vi "UiControls_b2g2.vi"() -> ()   [LabVIEW 2011]
uses:
  Output - Cluster b2g2.ctl
  Input - Cluster b2g2.ctl
panel:
  out "Array":errorcluster[](array[cluster])
  in  "Tab Control":enum32{"auto", "manual", "timetable", "tools"}(tab)
  in  "circulation ctl":bool
  in  "off [min]":u8=10 step=1 format="%#_3g"
  in  "on [min]":u8=10 step=1 format="%#_3g"
  in  "level ctl":bool
  in  "pressure ctl":bool
  in  "dosage ctl":bool
  in  "temp. ctl":bool
  in  "setpoint [l]":sgl=2.4 min=0 max=5 step=0.1 format="%.1g"
  in  "setpoint [bar]":sgl=10.0 min=0 max=10 step=0.1 format="%.1g"
  in  "flow [l/min]":sgl=1.5 format="%.1g"
  in  "volume [l]":sgl=1.0 step=0.1 format="%.1g"
  in  "hysteresis [°C]":sgl=0.05 min=0.01 max=10 step=0.01 format="%.2g"
  in  "setpoint [°C]":sgl=37.0 min=0 max=100 step=0.1 format="%.1g"
  in  "Tank":enum32{"Tank 1", "Tank 2 (Flash)"}(radio) caption="source"
  in  "P-9":bool
  in  "V-34":bool
  in  "V-33":bool
  in  "V-13 [%]":u8=10 caption="opening [%]" max=100 step=1
  in  "V-15  [%]":u8 caption="opening [%]" max=100 step=1
  in  "P-4 Drehzahl  [%]":u8=50 caption="speed  [%]"
  in  "P-4":bool
  in  "HS-1":bool
  in  "Interval [ms]":u32=10 caption="interval [ms]" min=10 step=1
  in  "Target Log":bool caption="crio log"
  in  "V-35":bool
  in  "T-1 & T-2  \nlevel-monitoring":bool=TRUE
  in  "MR \nlevel-monitoring":bool=TRUE
  out "Volume T-2 [l]":dbl caption="T-2 [l]"
  out "Volume T-1 [l]":dbl caption="T-1 [l]"
  in  "on/off":bool caption="activate"
  in  "Zeitplan":string[][](table)=[["00:00", "0", "1", "1", "1,5"], ["01:00", "0", "1", "1", "1,5"], ["02:00", "0", "1", "1", "1,5"], ["03:00", "0", "1", "1", "1,5"], ["04:00", "0", "1", "1", "1,5"], ["05:00", "0", "1", "1", "1,5"], ["06:00", "0", "1", "1", "1,5"], ["07:00", "0", "1", "1", "1,5"], ["08:00", "0", "1", "1", "1,5"], ["09:00", "0", "1", "1", "1,5"], ["10:00", "0", "1", "1", "1,5"], ["11:00", "0", "1", "1", "1,5"], ["12:00", "0", "1", "1", "1,5"], ["13:00", "0", "1", "1", "1,5"], ["14:00", "0", "1", "1", "1,5"], ["15:00", "0", "1", "1", "1,5"], ["16:00", "0", "1", "1", "1,5"], ["17:00", "0", "1", "1", "1,5"], ["18:00", "0", "1", "1", "1,5"], ["19:00", "0", "1", "1", "1,5"], ["20:00", "0", "1", "1", "1,5"], ["21:00", "0", "1", "1", "1,5"], ["22:00", "0", "1", "1", "1,5"], ["23:00", "0", "1", "1", "1,5"]]
  in  "stop":bool caption="stop crio"
  out "pc":timestamp
  out "crio":timestamp
  in  "load/save":enum16{"Load", "Save"}(ring)
  in  "enter":bool
  in  "config file":path caption="path"
  # "accumulated \nvolume"
  # "timestamp"
  # "configurtaion file"
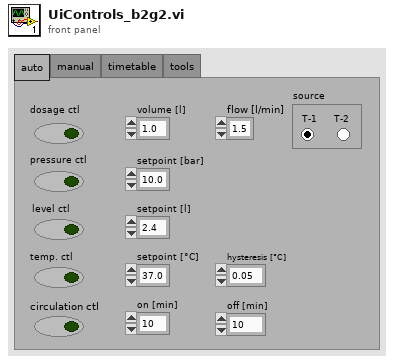
[diagram p1: front panel]
types:
  T1 = typedef "Output - Cluster b2g2.ctl" = cluster{"DFS-1 [dl]":u64, "FS-3 [l]":dbl, "DFS-1 [l/min]":dbl, "DS-1 [bar]":dbl, "V-10 ZU":bool, "V-14 ZU":bool, "FS-1 [l]":dbl, "FS-2 [l]":dbl, "TS-4 [°C]":dbl, "HS-1":bool, "V-13 [%]":u8, "V-15 [%]":u8, "P-4 [%]":u8, "Dosierung":bool, "MR Max Füllstand":bool, "MR Min Füllstand":bool, "Dosiermenge [l]":sgl, "V-14 AUF":bool, "V-10 AUF":bool, "T-1 Max Füllstand":bool, "T-1 Min Füllstand":bool, "T-2 Max Füllstand":bool, "T-2 Min Füllstand":bool, "pHS-1 [pH]":dbl, "P-4 RUN":bool, "V-33 AUF":bool, "V-33 ZU":bool, "V-34 AUF":bool, "V-34 ZU":bool, "P-4 ERR":bool, "TS-5 [°C]":dbl, "V-35 AUF":bool, "V-35 ZU":bool, "P-9 RUN":bool}
  T2 = typedef "Input - Cluster b2g2.ctl" = cluster{"V-13 [%]":u8, "V-15 [%]":u8, "Log-Target":bool, "P-4":bool, "P-4 Drehzahl [%]":u8, "Temperaturregelung":bool, "Überdruckregelung":bool, "Füllstandsregulierung":bool, "V-10":bool, "Log-Host":bool, "V-14":bool, "HS-1":bool, "Füllstand  P":sgl, "Füllstand I":sgl, "Füllstand D":sgl, "Füllstand Soll [l]":sgl, "Druck  P":sgl, "Druck I":sgl, "Druck D":sgl, "Druck Soll [bar]":sgl, "Temp Soll [°C]":sgl, "Dosierung":bool, "Dosiermenge [l]":sgl, "Dosiergeschw. [l/min]":sgl, "Tank":bool, "Hysterese [°C]":sgl, "MR Füllstandsüberwachung":bool, "Tank Füllstandsüberwachung":bool, "Log Target [ms]":u32, "Log Host [s]":u32, "Zirkulation EIN [min]":u8, "Zirkulation AUS [min]":u8, "Zirkulation":bool, "V-33":bool, "V-34":bool, "V-35":bool, "T1 Max Füllstand":bool, "T1 Min Füllstand":bool, "FS-1 [l]":sgl, "P-9":bool}
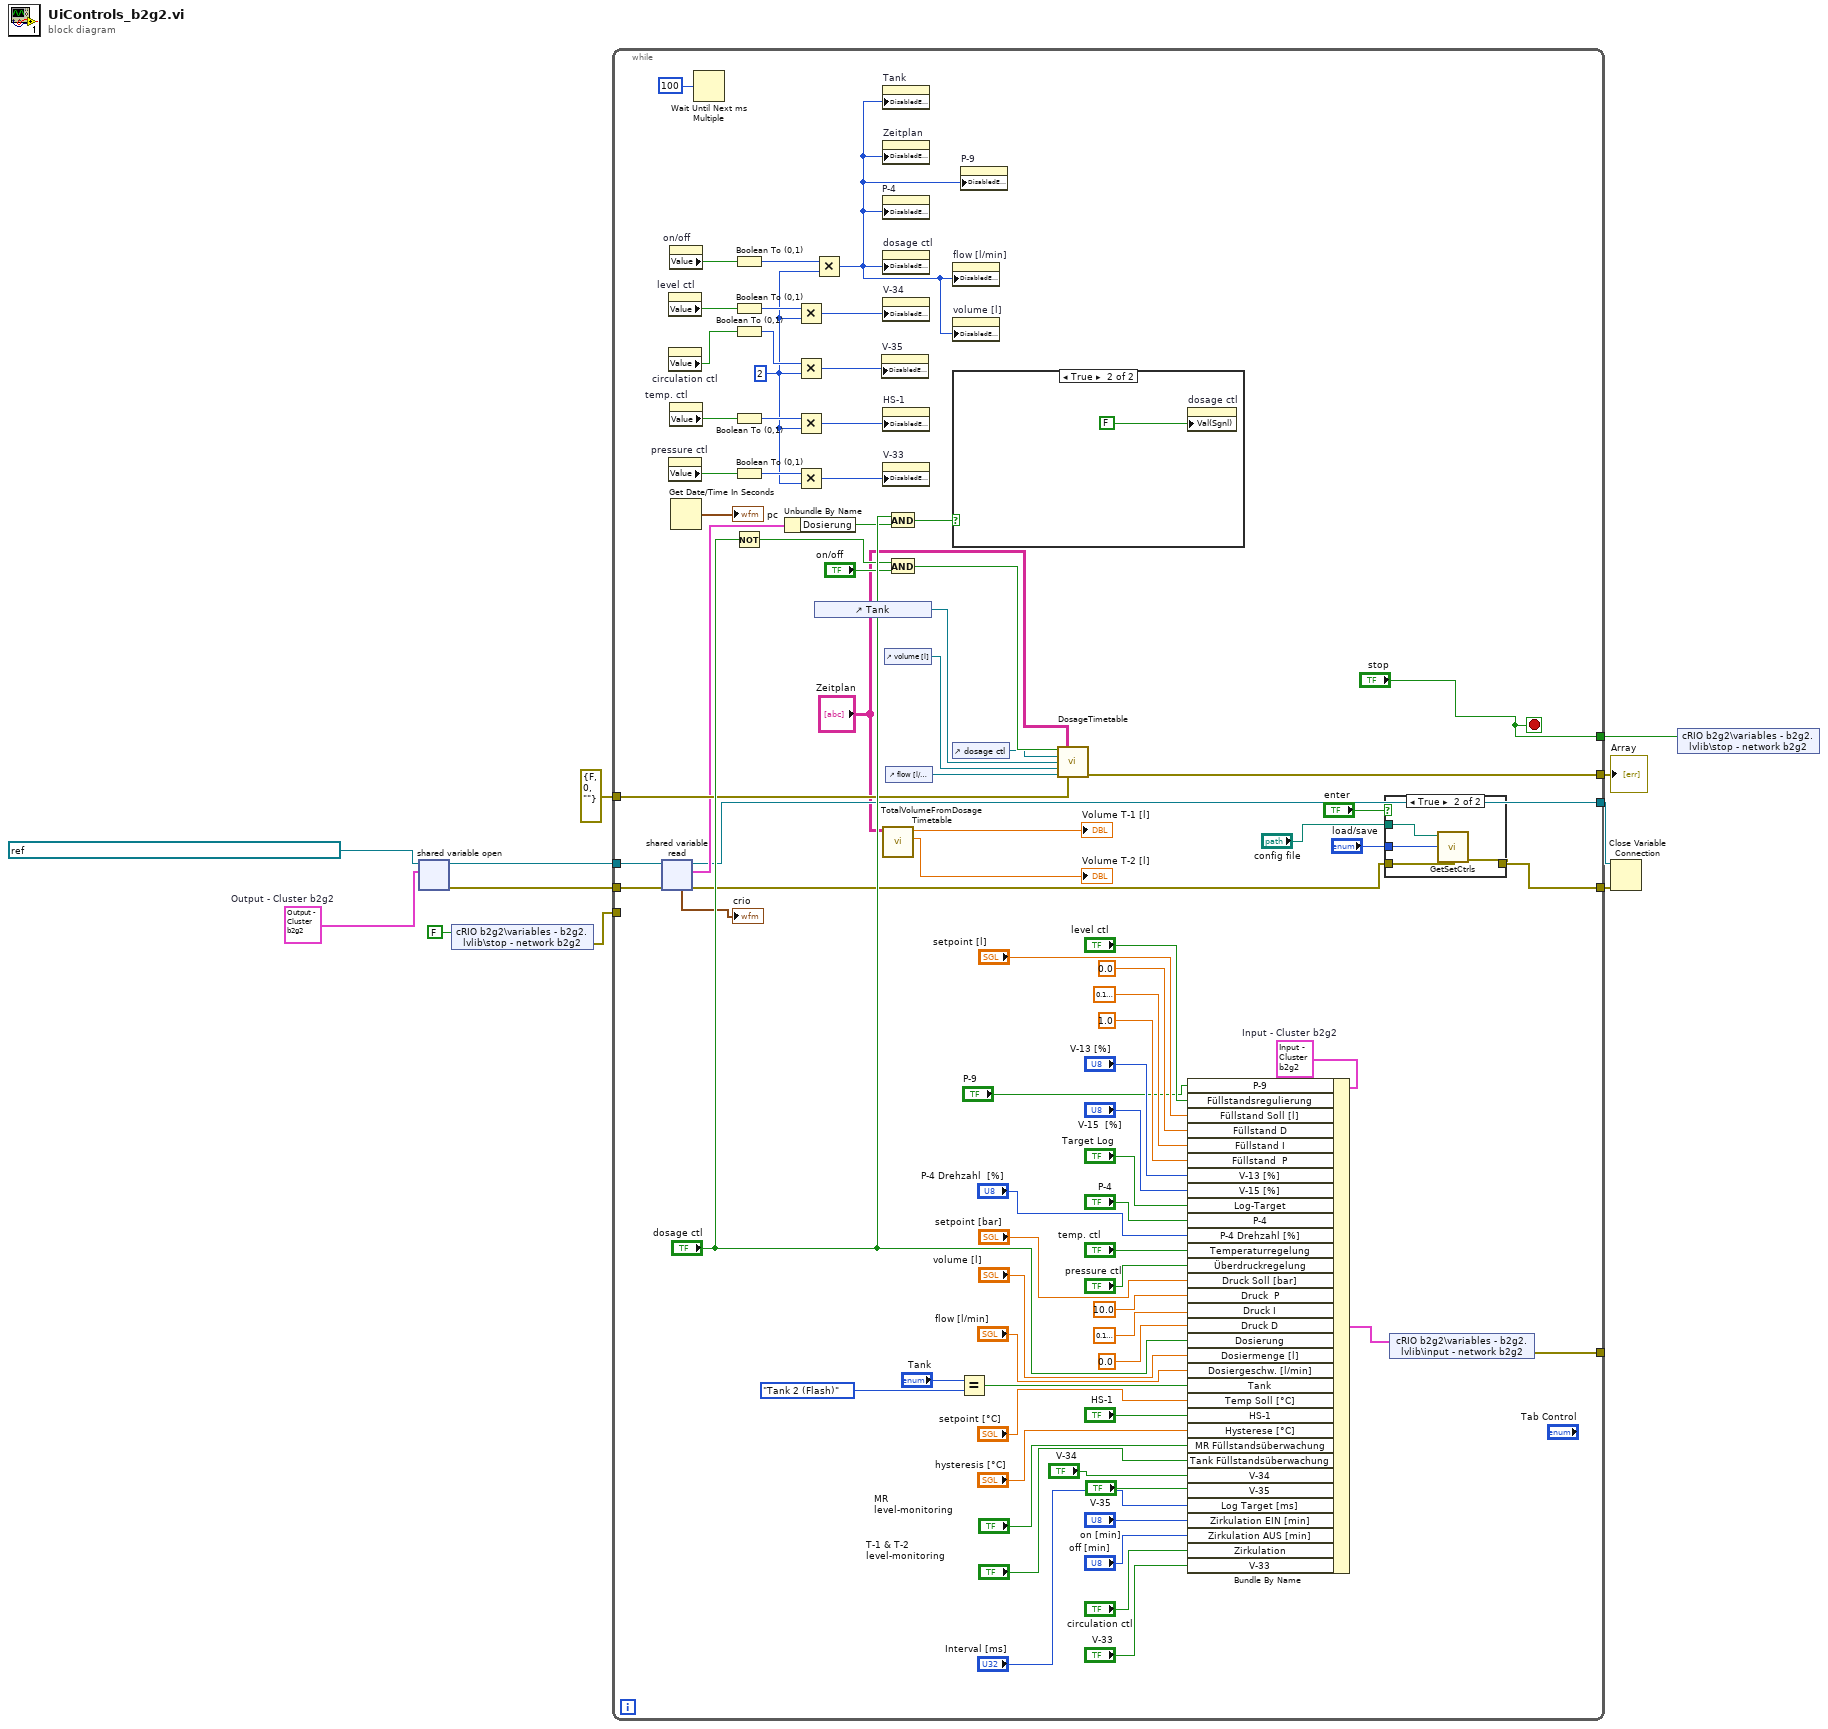
[diagram p0: block diagram]
diagram:
  w1 = T1 {"DFS-1 [dl]"=0, "FS-3 [l]"=0.0, "DFS-1 [l/min]"=0.0, "DS-1 [bar]"=0.0, "V-10 ZU"=FALSE, "V-14 ZU"=FALSE, "FS-1 [l]"=0.0, "FS-2 [l]"=0.0, "TS-4 [°C]"=0.0, "HS-1"=FALSE, "V-13 [%]"=0, "V-15 [%]"=0, "P-4 [%]"=0, "Dosierung"=FALSE, "MR Max Füllstand"=FALSE, "MR Min Füllstand"=FALSE, "Dosiermenge [l]"=0.0, "V-14 AUF"=FALSE, "V-10 AUF"=FALSE, "T-1 Max Füllstand"=FALSE, "T-1 Min Füllstand"=FALSE, "T-2 Max Füllstand"=FALSE, "T-2 Min Füllstand"=FALSE, "pHS-1 [pH]"=0.0, "P-4 RUN"=FALSE, "V-33 AUF"=FALSE, "V-33 ZU"=FALSE, "V-34 AUF"=FALSE, "V-34 ZU"=FALSE, "P-4 ERR"=FALSE, "TS-5 [°C]"=0.0, "V-35 AUF"=FALSE, "V-35 ZU"=FALSE, "P-9 RUN"=FALSE}  # Output - Cluster b2g2
  n1 = shared-variable-open(refnum<k21> "ni.var.psp://10.27.40.25/variables - b2g2/data - network b2g2" ("shared variable refnum in"), w1) -> (w5:refnum<k21>, w3:errorcluster)  [unwired: 2 in]
  n2 = shared-variable "cRIO b2g2\\variables - b2g2.lvlib\\stop - network b2g2"(FALSE ("stop - network")) -> (error out=w10:errorcluster)  [unwired: 1 in]
  n3 = while {
    tunnel: ["stop"] -> w11
    tunnel: w10 -> [_]
    tunnel: [w69] -> _
    tunnel: errorcluster {"status"=FALSE, "code"=0, "source"=""} ("error out") -> [w38]
    tunnel: [w32] -> w7
    tunnel: w5 -> [w30]
    tunnel: [w28] -> w4
    tunnel: w3 -> [w27]
    tunnel: [w15] -> w2
    stop <- "stop" stop-if-true
    w89 = T2 {"V-13 [%]"=0, "V-15 [%]"=0, "Log-Target"=FALSE, "P-4"=FALSE, "P-4 Drehzahl [%]"=0, "Temperaturregelung"=FALSE, "Überdruckregelung"=FALSE, "Füllstandsregulierung"=FALSE, "V-10"=FALSE, "Log-Host"=FALSE, "V-14"=FALSE, "HS-1"=FALSE, "Füllstand  P"=0.0, "Füllstand I"=0.0, "Füllstand D"=0.0, "Füllstand Soll [l]"=0.0, "Druck  P"=0.0, "Druck I"=0.0, "Druck D"=0.0, "Druck Soll [bar]"=0.0, "Temp Soll [°C]"=0.0, "Dosierung"=FALSE, "Dosiermenge [l]"=0.0, "Dosiergeschw. [l/min]"=0.0, "Tank"=FALSE, "Hysterese [°C]"=0.0, "MR Füllstandsüberwachung"=FALSE, "Tank Füllstandsüberwachung"=FALSE, "Log Target [ms]"=0, "Log Host [s]"=0, "Zirkulation EIN [min]"=0, "Zirkulation AUS [min]"=0, "Zirkulation"=FALSE, "V-33"=FALSE, "V-34"=FALSE, "V-35"=FALSE, "T1 Max Füllstand"=FALSE, "T1 Min Füllstand"=FALSE, "FS-1 [l]"=0.0, "P-9"=FALSE}  # Input - Cluster b2g2
    w44 = i16 2 ("y")
    n4 = shared-variable-read(w30, w27) -> (w28:refnum<k21>, w16:errorcluster, w29:T1, →"crio":timestamp)
    n5 = property on="level ctl" class="Bool (strict)"() -> ("Value"=w45:bool)  [unwired: 2 in, 2 out]
    n6 = property on="circulation ctl" class="Bool (strict)"() -> ("Value"=w47:bool)  [unwired: 2 in, 2 out]
    n7 = property on="pressure ctl" class="Bool (strict)"() -> ("Value"=w46:bool)  [unwired: 2 in, 2 out]
    n8 = property on="on/off" class="Bool (strict)"() -> ("Value"=w55:bool)  [unwired: 2 in, 2 out]
    n9 = property on="temp. ctl" class="Bool (strict)"() -> ("Value"=w52:bool)  [unwired: 2 in, 2 out]
    n10 = Get Date/Time In Seconds() -> (seconds since 1Jan1904=→"pc":timestamp)
    n11 = Wait Until Next ms Multiple(millisecond multiple=u32 100) -> ()  [unwired: 1 out]
    n12 = Boolean To (0,1)(Boolean=w55) -> (0, 1=w54:i16)
    n13 = Boolean To (0,1)(Boolean=w45) -> (0, 1=w50:i16)
    n14 = Boolean To (0,1)(Boolean=w47) -> (0, 1=w48:i16)
    n15 = Boolean To (0,1)(Boolean=w52) -> (0, 1=w53:i16)
    n16 = Boolean To (0,1)(Boolean=w46) -> (0, 1=w49:i16)
    n17 = Not(x="dosage ctl") -> (.not. x?=w57:bool)
    n18 = Unbundle By Name(w29) -> ("Dosierung"=w31:bool)
    n19 = Multiply(x=w50, y=w44) -> (x*y=w42:i16)
    n20 = Multiply(x=w48, y=w44) -> (x*y=w19:i16)
    n21 = Multiply(x=w53, y=w44) -> (x*y=w51:i16)
    n22 = Multiply(x=w49, y=w44) -> (x*y=w43:i16)
    n23 = Multiply(x=w54, y=w44) -> (x*y=w12:i16)
    n24 = control-ref of="Tank"() -> (w35:refnum<vi>)
    n25 = property on="V-35" class="Bool (strict)"("DisabledEnum"=w19) -> ()  [unwired: 2 in, 2 out]
    n26 = property on="Tank" class="RadioBtnsControl (strict)"("DisabledEnum"=w12) -> ()  [unwired: 2 in, 2 out]
    n27 = property on="Zeitplan" class="Tbl (strict)"("DisabledEnum"=w12) -> ()  [unwired: 2 in, 2 out]
    n28 = property on="P-4" class="Bool (strict)"("DisabledEnum"=w12) -> ()  [unwired: 2 in, 2 out]
    n29 = property on="dosage ctl" class="Bool (strict)"("DisabledEnum"=w12) -> ()  [unwired: 2 in, 2 out]
    n30 = property on="V-34" class="Bool (strict)"("DisabledEnum"=w42) -> ()  [unwired: 2 in, 2 out]
    n31 = property on="HS-1" class="Bool (strict)"("DisabledEnum"=w51) -> ()  [unwired: 2 in, 2 out]
    n32 = property on="V-33" class="Bool (strict)"("DisabledEnum"=w43) -> ()  [unwired: 2 in, 2 out]
    n33 = call "TotalVolumeFromDosageTimetable.vi"("Zeitplan"="Zeitplan") -> ("Volume T-2 [l]"=→"Volume T-2 [l]":dbl, "Volume T-1 [l]"=→"Volume T-1 [l]":dbl)  [unwired: 9 in]
    n34 = control-ref of="volume [l]"() -> (w34:refnum<vi>)
    n35 = control-ref of="flow [l/min]"() -> (w33:refnum<vi>)
    n36 = And(x="dosage ctl", y=w31) -> (x .and. y?=w63:bool)
    n37 = And(x=w57, y="on/off") -> (x .and. y?=w37:bool)
    n38 = property on="flow [l/min]" class="DigNum (strict)"("DisabledEnum"=w12) -> ()  [unwired: 2 in, 2 out]
    n39 = property on="volume [l]" class="DigNum (strict)"("DisabledEnum"=w12) -> ()  [unwired: 2 in, 2 out]
    n40 = case shown="True" w63 {
      frame False {
      }
      frame True {
        n41 = property on="dosage ctl" class="Bool (strict)"("Val(Sgnl)"=FALSE ("Value (Signaling)")) -> ()  [unwired: 2 in, 2 out]
      }
    }
    n42 = control-ref of="dosage ctl"() -> (w36:refnum<vi>)
    n43 = Equal?(x="Tank", y=enum32{"Tank 1", "Tank 2 (Flash)"}."Tank 2 (Flash)") -> (x = y?=w60:bool)
    n44 = property on="P-9" class="Bool (strict)"("DisabledEnum"=w12) -> ()  [unwired: 2 in, 2 out]
    n45 = call "DosageTimetable.vi"("enable"=w37, "timetable"="Zeitplan", "dosage"=w36, "tank"=w35, "volume"=w34, "flowrate"=w33, "error in"=w38) -> ("error out"=w32:errorcluster[])  [unwired: 8 in]
    n46 = Bundle By Name(cluster=w89, "P-9"="P-9", "Füllstandsregulierung"="level ctl", "Füllstand Soll [l]"="setpoint [l]", "Füllstand D"=sgl 0.0 ("D 2"), "Füllstand I"=sgl 0.1 ("I 2"), "Füllstand  P"=sgl 1.0 ("P 2"), "V-13 [%]"="V-13 [%]", "V-15 [%]"="V-15  [%]", "Log-Target"="Target Log", "P-4"="P-4", "P-4 Drehzahl [%]"="P-4 Drehzahl  [%]", "Temperaturregelung"="temp. ctl", "Überdruckregelung"="pressure ctl", "Druck Soll [bar]"="setpoint [bar]", "Druck  P"=sgl 10.0 ("P"), "Druck I"=sgl 0.1 ("I"), "Druck D"=sgl 0.0 ("D"), "Dosierung"="dosage ctl", "Dosiermenge [l]"="volume [l]", "Dosiergeschw. [l/min]"="flow [l/min]", "Tank"=w60, "Temp Soll [°C]"="setpoint [°C]", "HS-1"="HS-1", "Hysterese [°C]"="hysteresis [°C]", "MR Füllstandsüberwachung"="MR \nlevel-monitoring", "Tank Füllstandsüberwachung"="T-1 & T-2  \nlevel-monitoring", "V-34"="V-34", "V-35"="V-35", "Log Target [ms]"="Interval [ms]", "Zirkulation EIN [min]"="on [min]", "Zirkulation AUS [min]"="off [min]", "Zirkulation"="circulation ctl", "V-33"="V-33") -> (w70:T2)
    n47 = case shown="True" "enter" {
      tunnel: w16 -> [w93 w97]
      tunnel: [w93 w96] -> w15
      tunnel: "load/save" -> [_ w95]
      tunnel: "config file" -> [_ w94]
      frame False {
      }
      frame True {
        n48 = call "GetSetCtrls.vi"("error in (no error)"=w97, "Function (Load)"=w95, "Ini file (empty)"=w94) -> ("error out"=w96:errorcluster)  [unwired: 8 in]
      }
    }
    n49 = shared-variable "cRIO b2g2\\variables - b2g2.lvlib\\input - network b2g2"(w70) -> (error out=w69:errorcluster)  [unwired: 1 in]
  }
  "Array" <- w7
  n50 = Close Variable Connection(8:w2, 11:w4) -> ()  [unwired: 1 out]
  n51 = shared-variable "cRIO b2g2\\variables - b2g2.lvlib\\stop - network b2g2"(w11) -> ()  [unwired: 1 in, 1 out]
